vi "GetTorqueWfmByName.vi"(8 "error in (no error)":errorcluster, 10 "Channel Name":string, 11 "Torque Waveform in":waveform(sgl)) -> (0 "error out":errorcluster, 1 "Torque Waveform out":waveform(sgl), 2 "Found?":bool)   [LabVIEW 2017, in "McsaUtilities.lvlib"]
uses:
  <vilib>/addons/InsightCM/Utilities/MCSA/McsaUtilities.lvlib
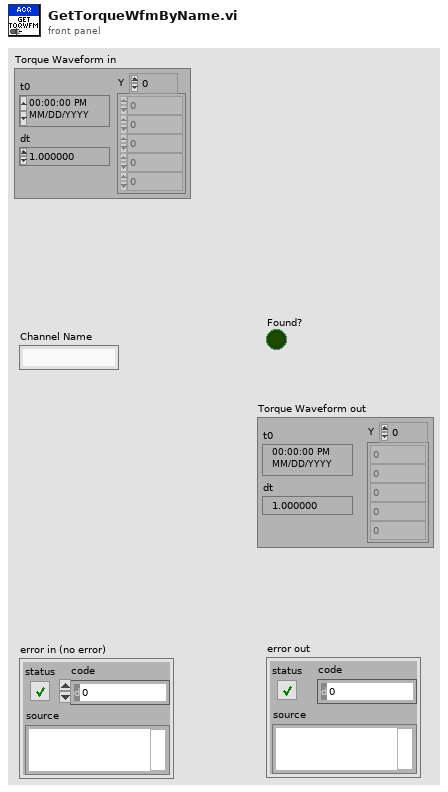
[diagram p1: front panel]
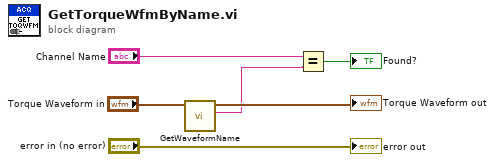
[diagram p0: block diagram]
diagram:
  n1 = call <vilib>:"GetWaveformName.vi"("waveform in"="Torque Waveform in") -> ("channel name"=w1:string, "waveform out"=→"Torque Waveform out":waveform(sgl))  [unwired: 9 in]
  n2 = Equal?(x="Channel Name", y=w1) -> (x = y?=→"Found?":bool)
  "error out" <- "error in (no error)"
